vi "ex5_moje.vi"() -> ()   [LabVIEW 2022 SP3]
panel:
  out "XY Graph":cluster{i32[], dbl[]}[](graph)
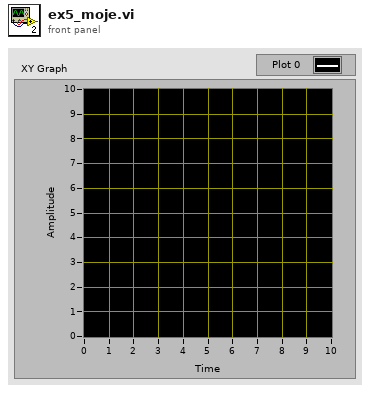
[diagram p1: front panel]
types:
  T1 = enum16{"big-endian, network order", "native, host order", "little-endian"}
  T2 = enum16{"open", "replace", "create", "open or create", "replace or create", "replace or create with confirmation"}
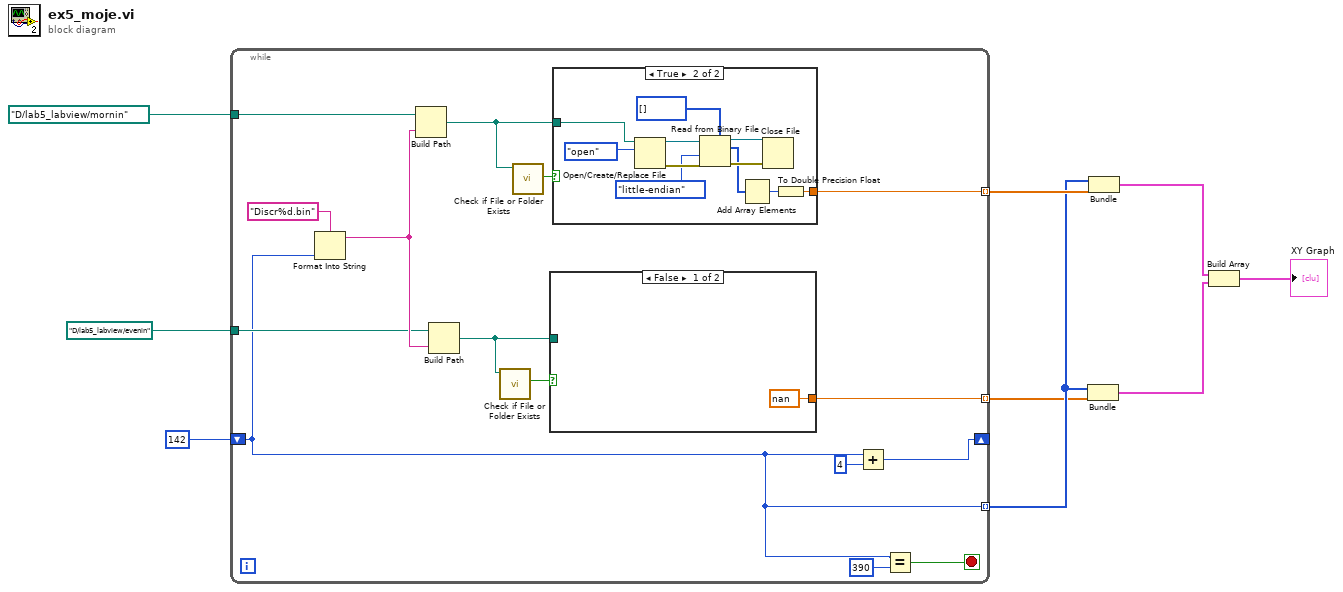
[diagram p0: block diagram]
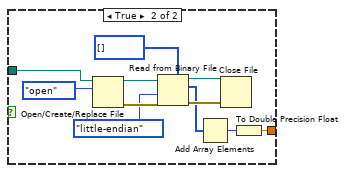
[diagram p2: hidden frame]
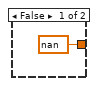
[diagram p3: hidden frame]
diagram:
  n1 = while {
    tunnel: path "D:/lab5_labview/mornin" ("file path (use dialog)") -> [w24]
    shift-right: [w14] -> _
    shift-left: 142 -> [w11]
    tunnel: [w20] -> w6 mode=indexing
    tunnel: path "D:/lab5_labview/evenin" ("file (use dialog)") -> [w18]
    tunnel: [w11] -> w5 mode=indexing
    tunnel: [w10] -> w4 mode=indexing
    stop <- w12 stop-if-true
    n2 = Format Into String(format string="Discr%d.bin", w11) -> (resulting string=w19:string)  [unwired: 2 in, 1 out]
    n3 = Build Path(base path=w24, name or relative path=w19) -> (appended path=w23:path)
    n4 = Build Path(base path=w18, name or relative path=w19) -> (appended path=w16:path)
    n5 = call <vilib>:"Check if File or Folder Exists.vi"("path"=w16) -> ("file or folder exists?"=w17:bool)  [unwired: 8 in, 2 out]
    n6 = call <vilib>:"Check if File or Folder Exists.vi"("path"=w23) -> ("file or folder exists?"=w22:bool)  [unwired: 8 in, 2 out]
    n7 = case shown="False" w17 {
      tunnel: w16 -> [_ w27]
      tunnel: [nan w26] -> w10
      frame False {
      }
      frame True {
        n8 = Open/Create/Replace File(file path (use dialog)=w27, operation (0:open)=T2."open") -> (refnum out=w35:refnum<file>, error out=w34:errorcluster)  [unwired: 4 in, 1 out]
        n9 = Read from Binary File(5:u32[] [] ("array"), 8:w34, 9:T1."little-endian" ("byte order (0:big-endian, network order)"), 11:w35) -> (0:w30:errorcluster, 2:w29:u32[], 3:w31:refnum<file>)  [unwired: 2 in, 1 out]
        n10 = Add Array Elements(numeric array=w29) -> (sum=w28:u32)
        n11 = Close File(refnum=w31, error in=w30) -> ()  [unwired: 2 out]
        n12 = To Double Precision Float(number=w28) -> (double precision float=w26:dbl)
      }
    }
    n13 = case shown="True" w22 {
      tunnel: w23 -> [_ w47]
      tunnel: [nan w38] -> w20
      frame False {
      }
      frame True {
        n14 = Open/Create/Replace File(file path (use dialog)=w47, operation (0:open)=T2."open") -> (refnum out=w46:refnum<file>, error out=w45:errorcluster)  [unwired: 4 in, 1 out]
        n15 = Read from Binary File(5:u32[] [] ("array"), 8:w45, 9:T1."little-endian" ("byte order (0:big-endian, network order)"), 11:w46) -> (0:w41:errorcluster, 2:w40:u32[], 3:w42:refnum<file>)  [unwired: 2 in, 1 out]
        n16 = Add Array Elements(numeric array=w40) -> (sum=w39:u32)
        n17 = Close File(refnum=w42, error in=w41) -> ()  [unwired: 2 out]
        n18 = To Double Precision Float(number=w39) -> (double precision float=w38:dbl)
      }
    }
    n19 = Add(x=w11, y=4) -> (x+y=w14:i32)
    n20 = Equal?(x=w11, y=390) -> (x = y?=w12:bool)
  }
  n21 = Bundle(w5, w4) -> (w2:cluster{i32[], dbl[]})  [unwired: 1 in]
  n22 = Bundle(w5, w6) -> (w3:cluster{i32[], dbl[]})  [unwired: 1 in]
  n23 = Build Array(w3, w2) -> (→"XY Graph":cluster{i32[], dbl[]}[])
